vi "Merge Arrays.vi"(9 "Coerce window width":dbl, 10 "New Array":dbl[](array[numeric]), 11 "Old Array":dbl[](array[numeric])) -> (3 "New Array out":dbl[](array[numeric]))   [LabVIEW 2016]
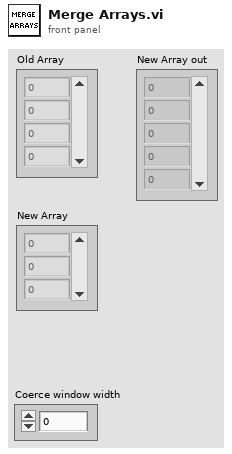
[diagram p1: front panel]
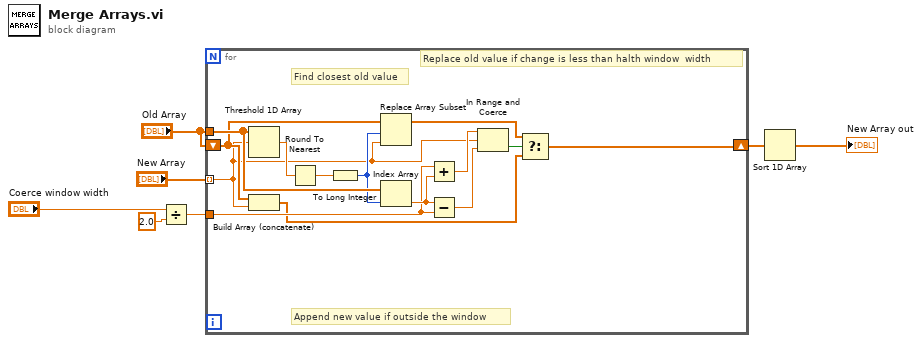
[diagram p0: block diagram]
diagram:
  n1 = Divide(x="Coerce window width", y=2.0) -> (x/y=w3:dbl)
  n2 = for {
    tunnel: "New Array" -> [w10] mode=indexing
    shift-right: [w8] -> w2
    shift-left: "Old Array" -> [w12]
    tunnel: "Old Array" -> [w19]
    tunnel: w3 -> [w16]
    # "Append new value if outside the window"
    # "Find closest old value"
    # "Replace old value if change is less than halth window  width"
    n3 = Threshold 1D Array(2:w10, 3:w19) -> (0:w21:dbl)  [unwired: 1 in]
    n4 = Build Array (concatenate)(w12, w10) -> (w9:dbl[])
    n5 = Round To Nearest(number=w21) -> (nearest integer value=w20:dbl)
    n6 = To Long Integer(number=w20) -> (32bit integer=w11:i32)
    n7 = Replace Array Subset(array=w12, new element=w10, index=w11) -> (w13:dbl[])
    n8 = Index Array(array=w19, index=w11) -> (element=w17:dbl)
    n9 = Add(x=w16, y=w17) -> (x+y=w18:dbl)
    n10 = Subtract(x=w17, y=w16) -> (x-y=w15:dbl)
    n11 = In Range and Coerce(upper limit=w18, x=w10, lower limit=w15) -> (In Range?=w14:bool)  [unwired: 1 out]
    n12 = Select(t=w13, s=w14, f=w9) -> (s? t:f=w8:dbl[])
  }
  n13 = Sort 1D Array(array=w2) -> (sorted array=→"New Array out":dbl[])
